vi "ShowDicomValues.vi"(8 "error in (no error)":errorcluster, 11 "Array":string[][](array[string])) -> (0 "error out":errorcluster)   [LabVIEW 2013, in "main.lvlib"]
uses:
  main.lvlib
panel:
  out "dicomValues Multicolumn Listbox":i32(listbox) caption="Multicolumn Listbox"
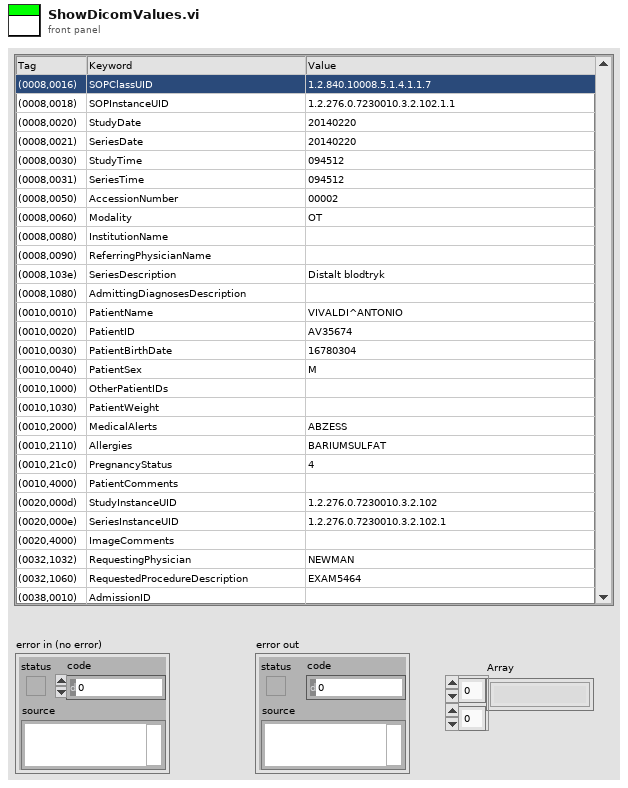
[diagram p1: front panel]
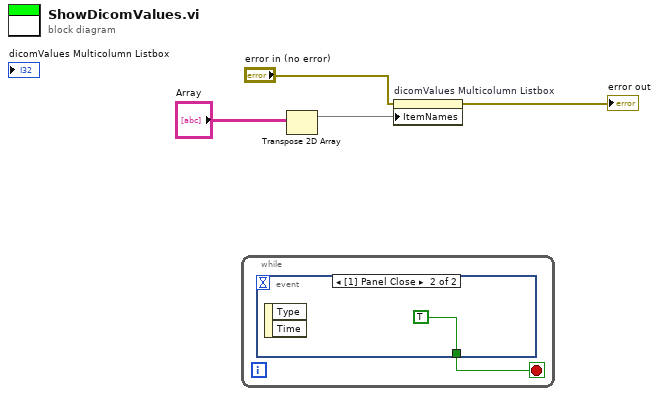
[diagram p0: block diagram]
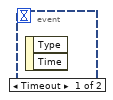
[diagram p2: hidden frame]
diagram:
  n1 = while {
    stop <- w5 stop-if-true
    n2 = event shown="[1] Panel Close" {
      selector: _ -> [_ _]
      dyn-events: _ -> [_ _]
      timeout: _ -> [_ _]
      tunnel: [_ TRUE] -> w5
      event Timeout {
        n3 = event-data() -> ()  [unwired: 1 in, 2 out]
      }
      event Panel Close {
        n4 = event-data() -> ()  [unwired: 1 in, 2 out]
      }
    }
  }
  n5 = Transpose 2D Array(2D array="Array") -> (transposed array=w4:string[][])
  n6 = property on="dicomValues Multicolumn Listbox" class="MCListbox (strict)"(error in="error in (no error)", "ItemNames"=w4) -> (error out=→"error out":errorcluster)  [unwired: 1 in, 1 out]
